vi "Sync_Write(one instruction packet).vi"(1 "ID&DEG_code&\nSpeed_code":u8[](array[numeric]), 2 "Actuator Number":i32=4) -> (0 "function return":i32)   [LabVIEW 2017]
uses:
  <userlib>/dynamixel/dynamixel.lvlib
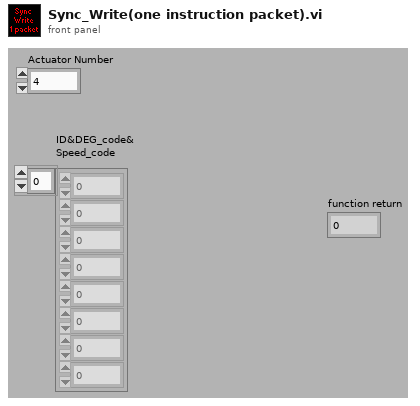
[diagram p1: front panel]
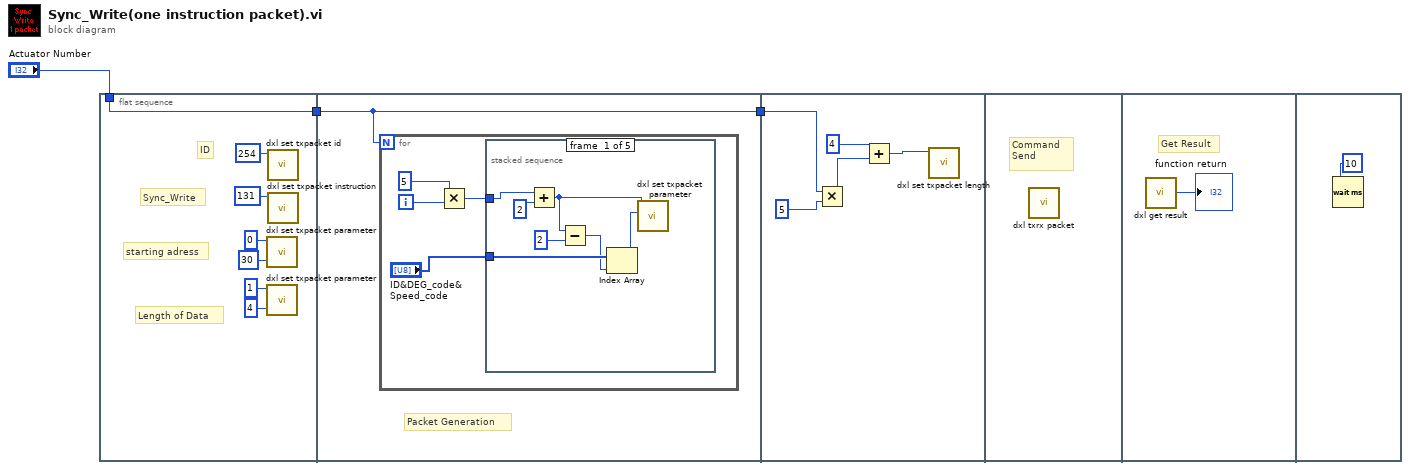
[diagram p0: block diagram]
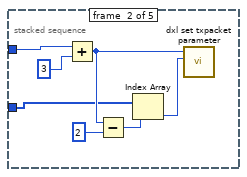
[diagram p2: hidden frame]
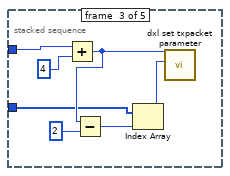
[diagram p3: hidden frame]
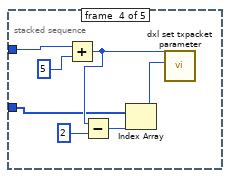
[diagram p4: hidden frame]
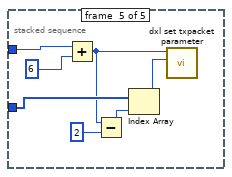
[diagram p5: hidden frame]
diagram:
  n1 = flat-sequence {
    tunnel: "Actuator Number" -> [w4]
    tunnel: [w4] -> w2
    tunnel: w2 -> [w11]
    tunnel: [w11] -> w1
    tunnel: w1 -> [w51]
    frame #0 {
      # "Length of Data"
      # "starting adress"
      # "Sync_Write"
      # "ID"
      n2 = call <userlib>:"dxl set txpacket parameter.vi"("value"=30, "index"=0) -> ()  [unwired: 10 in]
      n3 = call <userlib>:"dxl set txpacket parameter.vi"("value"=4, "index"=1) -> ()  [unwired: 10 in]
      n4 = call <userlib>:"dxl set txpacket id.vi"("id"=254) -> ()  [unwired: 11 in]
      n5 = call <userlib>:"dxl set txpacket instruction.vi"("instruction"=131) -> ()  [unwired: 11 in]
    }
    frame #1 {
      # "Packet Generation"
      n6 = for {
        N: w11 -> [_]
        i -> [w13]
        n7 = Multiply(x=5, y=w13) -> (x*y=w14:i32)
        n8 = stacked-sequence {
          tunnel: w14 -> [w22 w29 w36 w43 w50]
          tunnel: "ID&DEG_code&\nSpeed_code" -> [w20 w25 w31 w38 w47]
          frame #0 {
            n9 = Add(x=w22, y=2) -> (x+y=w18:i32)
            n10 = Subtract(x=w18, y=u8 2) -> (x-y=w17:i32)
            n11 = Index Array(array=w20, index=w17) -> (element=w16:u8)
            n12 = call <userlib>:"dxl set txpacket parameter.vi"("value"=w16, "index"=w18) -> ()  [unwired: 10 in]
          }
          frame #1 {
            n13 = Add(x=w29, y=3) -> (x+y=w26:i32)
            n14 = Subtract(x=w26, y=u8 2) -> (x-y=w24:i32)
            n15 = Index Array(array=w25, index=w24) -> (element=w23:u8)
            n16 = call <userlib>:"dxl set txpacket parameter.vi"("value"=w23, "index"=w26) -> ()  [unwired: 10 in]
          }
          frame #2 {
            n17 = Add(x=w36, y=4) -> (x+y=w32:i32)
            n18 = Subtract(x=w32, y=u8 2) -> (x-y=w33:i32)
            n19 = Index Array(array=w31, index=w33) -> (element=w30:u8)
            n20 = call <userlib>:"dxl set txpacket parameter.vi"("value"=w30, "index"=w32) -> ()  [unwired: 10 in]
          }
          frame #3 {
            n21 = Add(x=w43, y=5) -> (x+y=w39:i32)
            n22 = Subtract(x=w39, y=u8 2) -> (x-y=w40:i32)
            n23 = Index Array(array=w38, index=w40) -> (element=w37:u8)
            n24 = call <userlib>:"dxl set txpacket parameter.vi"("value"=w37, "index"=w39) -> ()  [unwired: 10 in]
          }
          frame #4 {
            n25 = Add(x=w50, y=6) -> (x+y=w45:i32)
            n26 = Subtract(x=w45, y=u8 2) -> (x-y=w46:i32)
            n27 = Index Array(array=w47, index=w46) -> (element=w44:u8)
            n28 = call <userlib>:"dxl set txpacket parameter.vi"("value"=w44, "index"=w45) -> ()  [unwired: 10 in]
          }
        }
      }
    }
    frame #2 {
      n29 = Multiply(x=w51, y=5 ("x")) -> (x*y=w53:i32)
      n30 = Add(x=4, y=w53) -> (x+y=w55:i32)
      n31 = call <userlib>:"dxl set txpacket length.vi"("length"=w55) -> ()  [unwired: 11 in]
    }
    frame #3 {
      # "Command\nSend"
      n32 = call <userlib>:"dxl txrx packet.vi"() -> ()  [unwired: 12 in]
    }
    frame #4 {
      # "Get Result"
      n33 = call <userlib>:"dxl get result.vi"() -> ("function return"=→"function return":i32)  [unwired: 11 in]
    }
    frame #5 {
      n34 = Wait (ms)(milliseconds to wait=u32 10 ("대기 시간(ms)")) -> ()  [unwired: 1 out]
    }
  }
